vi "Axial.vi"() -> ()   [LabVIEW 2017]
uses:
  <vilib>/Analysis/Matrix/Datatypes/RealMatrix.ctl
  <vilib>/Analysis/baseanly.llb/Mean (DBL).vi
  <vilib>/ULx/Create Channel.llb/ULx Create Channel (AI-Voltage-Basic).vi
  <vilib>/ULx/Timing.llb/ULx Timing (Sample Clock).vi
  <vilib>/ULx/Read.llb/ULx Read (Analog Wfm 1Chan NSamp).vi
  <vilib>/Utility/file.llb/Write Delimited Spreadsheet (DBL).vi
  <vilib>/Analysis/Matrix/Numeric/Conversions/Array To Matrix - RA.vi
  <vilib>/Analysis/NI_AALBase.lvlib
  <vilib>/Analysis/Matrix/NI_Matrix.lvlib
panel:
  out "Axial":cluster{"Weight":dbl[], "Voltage(Axial)":dbl[]}(graph)
  out "Rolling Moment":cluster{"Weight":dbl[], "Voltage(R.M.) ":dbl[]}(graph)
  out "S.F.":cluster{"Weight":dbl[], "Voltage(S.F.)":dbl[]}(graph)
  out "P.M.":cluster{"Weight":dbl[], "Voltage(P.M.)":dbl[]}(graph)
  out "n":cluster{"Weight":dbl[], "Voltage(n)":dbl[]}(graph)
  out "Normal":cluster{"Weight":dbl[], "Voltage(Normal)":dbl[]}(graph)
  out "Main Graph":cluster{"Weight":dbl[], "Main Voltage":dbl[]}(graph)
  out "Matrix Path Indicator":path
  in  "Record Matrix Path":path
  in  "Final Matrix":T1
  out "R.M. Sample Waveform":dbl[](graph)
  out "S.F. Sample Waveform":dbl[](graph)
  out "P.M. Sample Waveform":dbl[](graph)
  out "n Sample Waveform":dbl[](graph)
  out "Axial Force Sample Waveform":dbl[](graph)
  out "Normal Force Sample Waveform":dbl[](graph)
  out "Main Voltage":dbl[](array[numeric])
  out "Current Main Channel Calibration":string
  in  "Main Channel":string(combo)
  in  "Rolling Moment Physical Channel":refnum<k21>
  in  "S.F. Physical Channel":refnum<k21>
  in  "P.M. Physical Channel":refnum<k21>
  in  "n Physical Channel":refnum<k21>
  in  "Normal Force Physical Channel":refnum<k21>
  in  "minimum value":dbl=-5.0
  in  "maximum value":dbl=5.0
  in  "samples per channel":i32=100
  in  "sample mode":i32(ring) items=["FiniteSamples", "ContinuousSamples"]
  in  "rate":dbl=5000.0
  in  "Axial Force Physical Channel":refnum<k21>
  out "Voltage(R.M.)":dbl[](array[numeric])
  out "Voltage(S.F.)":dbl[](array[numeric])
  out "Voltage(P.M.)":dbl[](array[numeric])
  out "Voltage(n)":dbl[](array[numeric])
  out "Voltage(Normal)":dbl[](array[numeric])
  in  "Sample Button":bool
  in  "Add Weight":bool
  in  "Weight to be added":dbl
  out "Voltage(Axial)":dbl[](array[numeric])
  out "Weight":dbl[](array[numeric])
  in  "Clear Table":bool
  # "Channel and Sampling Selection"
  # "Interaction Plots\n\nPlots ALL SIX voltages,"
  # "Sample Waveform Graphs\n\nPlots all the data points onto a waveform graph in one sample Cycle, to see the range of noises and determine any bias in data."
  # "Voltages from EACH Channel\nRecords data from all six channels for each sample cycle. Each number represents the mean of all values from one sample cycle recorded by one channel."
  # "Final Matrix\nThe final matrix that records the data from calibration and overwrites itself every time one calibration cycle is performed."
  # "Weight"
  # "Normal Force"
  # "Axial Force"
  # "n"
  # "P.M."
  # "S.F."
  # "Rolling Moment"
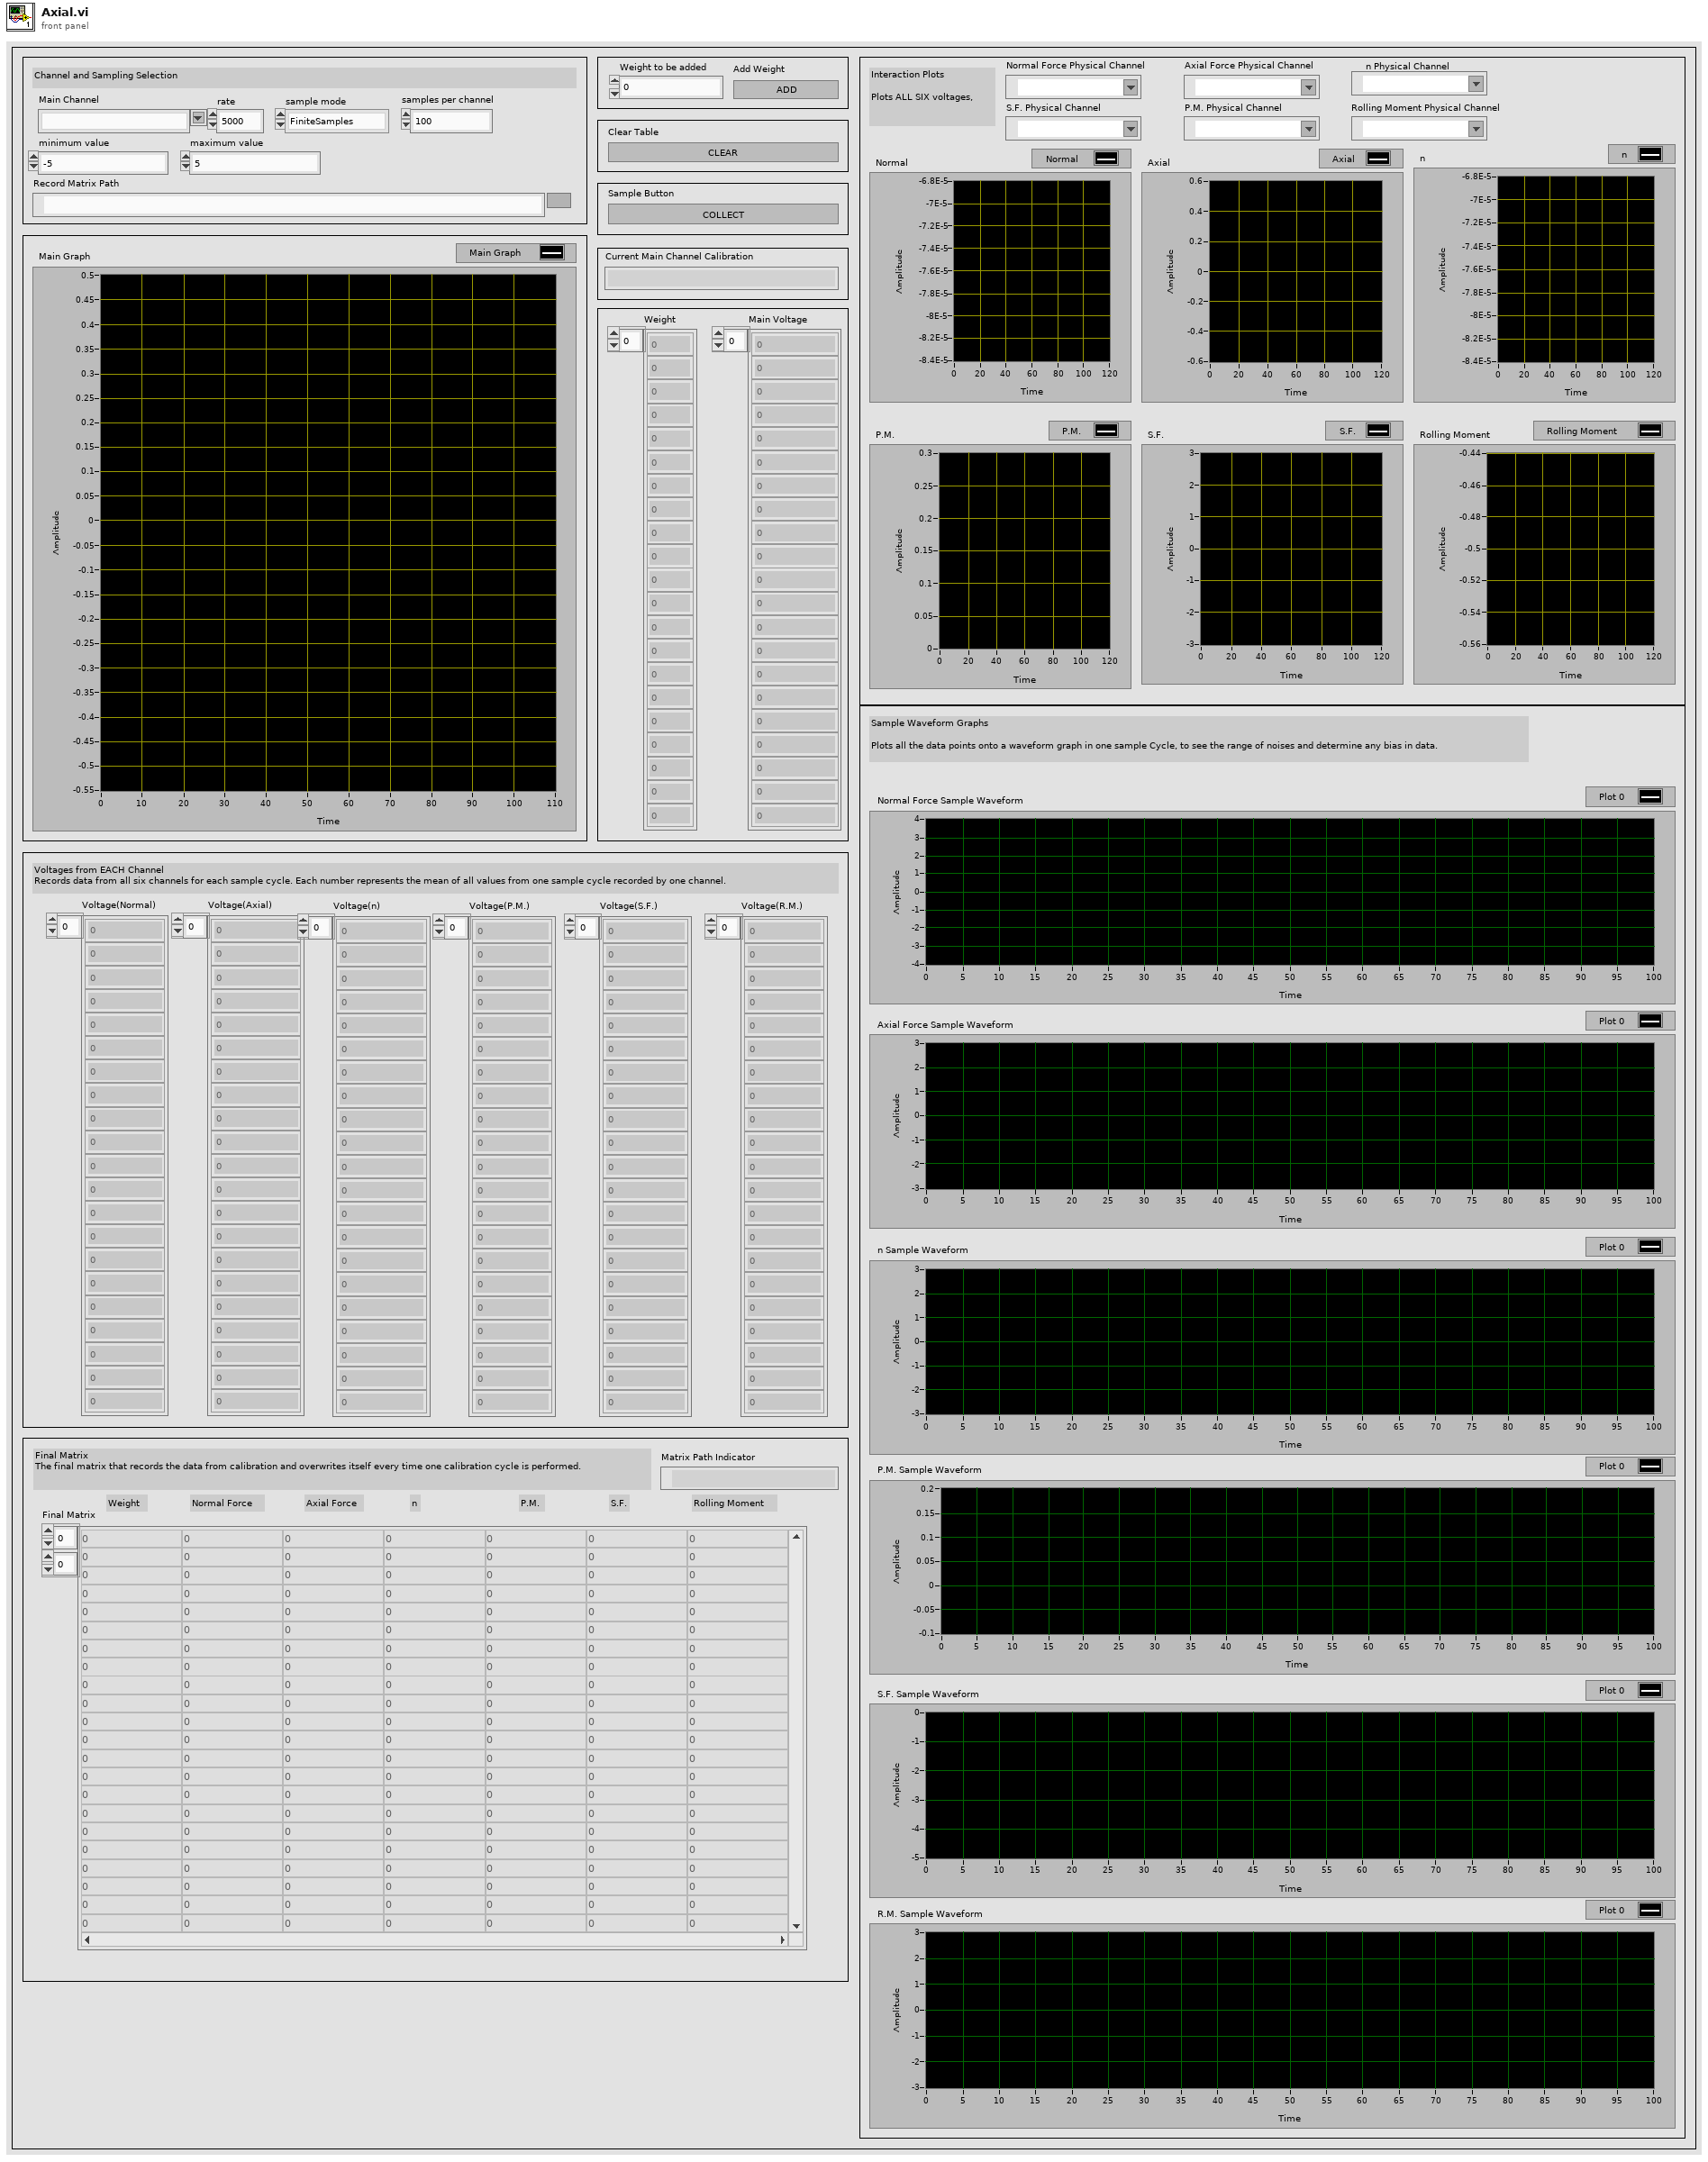
[diagram p1: front panel]
types:
  T1 = typedef "NI_Matrix.lvlib/RealMatrix.ctl" = dbl[][]
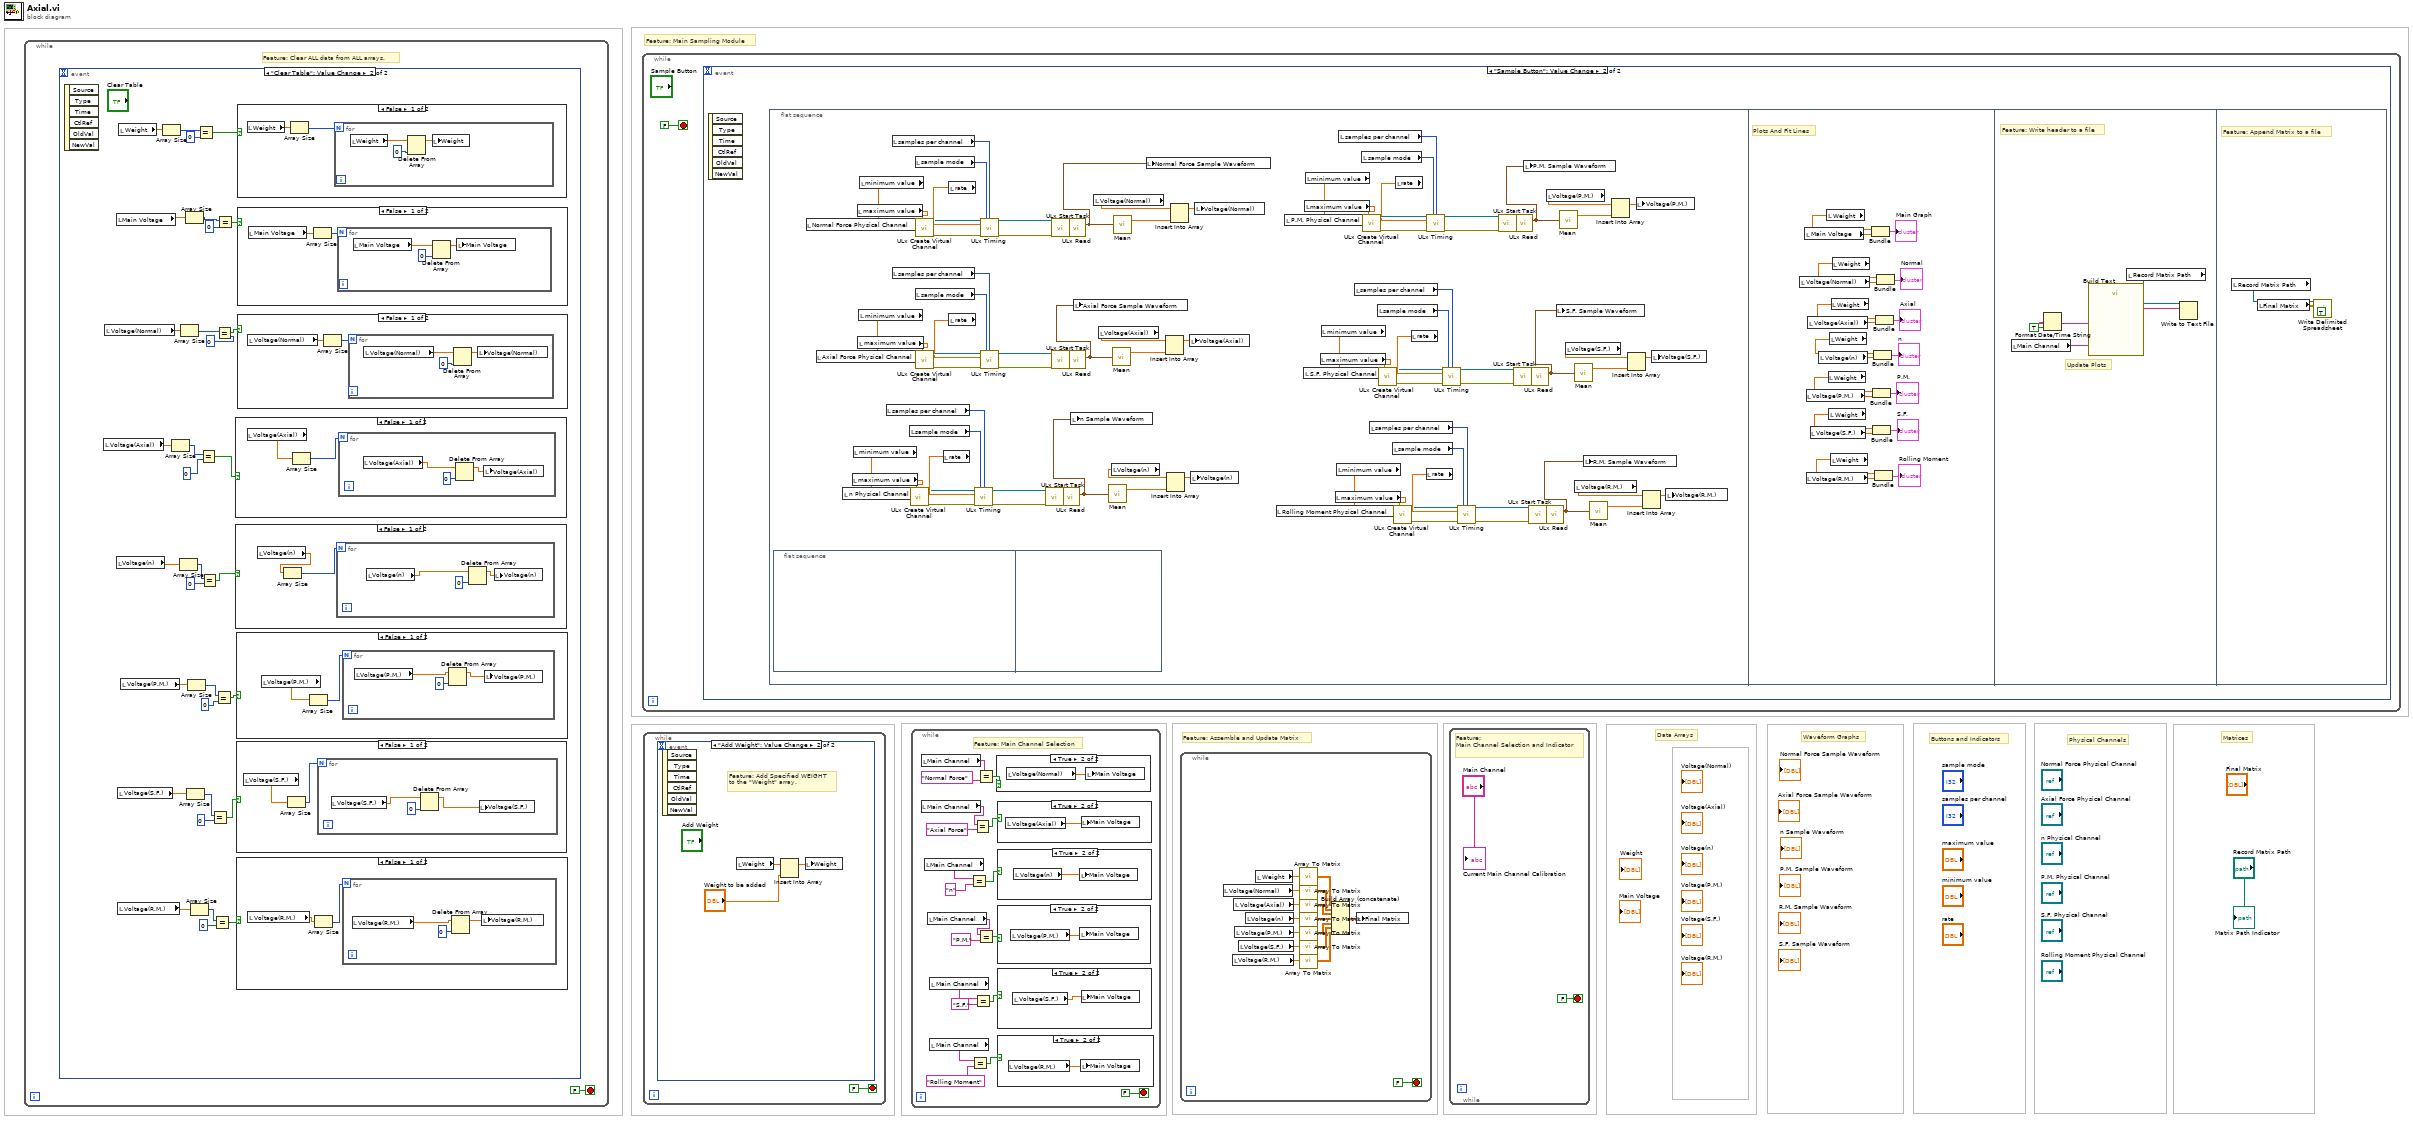
[diagram p0: block diagram]
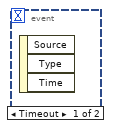
[diagram p8: hidden frame]
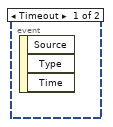
[diagram p17: hidden frame]
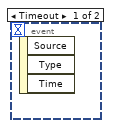
[diagram p18: hidden frame]
diagram:
  # "Matrices"
  # "Feature: Assemble and Update Matrix"
  # "Waveform Graphs"
  # "Physical Channels"
  # "Feature: Main Sampling Module"
  # "Data Arrays"
  # "Buttons and Indicators"
  n1 = while {
    stop <- FALSE stop-if-true
    # "Feature: Clear ALL data from ALL arrays."
    n2 = event shown="[1] \"Clear Table\": Value Change" {
      selector: _ -> [_ _]
      dyn-events: _ -> [_ _]
      timeout: _ -> [_ _]
      event Timeout {
        n3 = event-data() -> ()  [unwired: 1 in, 3 out]
      }
      event "Clear Table": Value Change {
        n4 = event-data() -> ()  [unwired: 1 in, 6 out]
        n5 = local read "Voltage(Axial)"() -> (w21:dbl[])
        n6 = local read "Voltage(Normal)"() -> (w24:dbl[])
        n7 = local read "Main Voltage"() -> (w30:dbl[])
        n8 = local read "Voltage(n)"() -> (w18:dbl[])
        n9 = local read "Voltage(S.F.)"() -> (w10:dbl[])
        n10 = local read "Voltage(R.M.)"() -> (w6:dbl[])
        n11 = local read "Weight"() -> (w31:dbl[])
        n12 = local read "Voltage(P.M.)"() -> (w13:dbl[])
        n13 = Array Size(array=w31) -> (size(s)=w34:i32)
        n14 = Array Size(array=w21) -> (size(s)=w22:i32)
        n15 = Array Size(array=w18) -> (size(s)=w17:i32)
        n16 = Array Size(array=w24) -> (size(s)=w25:i32)
        n17 = Array Size(array=w30) -> (size(s)=w29:i32)
        n18 = Array Size(array=w10) -> (size(s)=w9:i32)
        n19 = Array Size(array=w13) -> (size(s)=w14:i32)
        n20 = Array Size(array=w6) -> (size(s)=w5:i32)
        n21 = Equal?(x=w34, y=0) -> (x = y?=w32:bool)
        n22 = Equal?(x=w22, y=0) -> (x = y?=w19:bool)
        n23 = Equal?(x=w17, y=0) -> (x = y?=w15:bool)
        n24 = Equal?(x=w9, y=0) -> (x = y?=w7:bool)
        n25 = Equal?(x=w5, y=0) -> (x = y?=w4:bool)
        n26 = Equal?(x=w14, y=0) -> (x = y?=w11:bool)
        n27 = Equal?(x=w25, y=0) -> (x = y?=w26:bool)
        n28 = Equal?(x=w29, y=0) -> (x = y?=w27:bool)
        n29 = case shown="False" w19 {
          frame False {
            n30 = local read "Voltage(Axial)"() -> (w56:dbl[])
            n31 = Array Size(array=w56) -> (size(s)=w55:i32)
            n32 = for {
              N: w55 -> [_]
              n33 = local read "Voltage(Axial)"() -> (w59:dbl[])
              n34 = Delete From Array(array=w59, index=0) -> (array with subset deleted=w57:dbl[])  [unwired: 1 in, 1 out]
              n35 = local write "Voltage(Axial)"(w57) -> ()
            }
          }
          frame True {
          }
        }
        n36 = case shown="False" w15 {
          frame False {
            n37 = local read "Voltage(n)"() -> (w51:dbl[])
            n38 = Array Size(array=w51) -> (size(s)=w50:i32)
            n39 = for {
              N: w50 -> [_]
              n40 = local read "Voltage(n)"() -> (w54:dbl[])
              n41 = Delete From Array(array=w54, index=0) -> (array with subset deleted=w52:dbl[])  [unwired: 1 in, 1 out]
              n42 = local write "Voltage(n)"(w52) -> ()
            }
          }
          frame True {
          }
        }
        n43 = case shown="False" w11 {
          frame False {
            n44 = local read "Voltage(P.M.)"() -> (w46:dbl[])
            n45 = Array Size(array=w46) -> (size(s)=w45:i32)
            n46 = for {
              N: w45 -> [_]
              n47 = local read "Voltage(P.M.)"() -> (w49:dbl[])
              n48 = Delete From Array(array=w49, index=0) -> (array with subset deleted=w47:dbl[])  [unwired: 1 in, 1 out]
              n49 = local write "Voltage(P.M.)"(w47) -> ()
            }
          }
          frame True {
          }
        }
        n50 = case shown="False" w7 {
          frame False {
            n51 = local read "Voltage(S.F.)"() -> (w41:dbl[])
            n52 = Array Size(array=w41) -> (size(s)=w40:i32)
            n53 = for {
              N: w40 -> [_]
              n54 = local read "Voltage(S.F.)"() -> (w44:dbl[])
              n55 = Delete From Array(array=w44, index=0) -> (array with subset deleted=w43:dbl[])  [unwired: 1 in, 1 out]
              n56 = local write "Voltage(S.F.)"(w43) -> ()
            }
          }
          frame True {
          }
        }
        n57 = case shown="False" w4 {
          frame False {
            n58 = local read "Voltage(R.M.)"() -> (w35:dbl[])
            n59 = Array Size(array=w35) -> (size(s)=w36:i32)
            n60 = for {
              N: w36 -> [_]
              n61 = local read "Voltage(R.M.)"() -> (w39:dbl[])
              n62 = Delete From Array(array=w39, index=0) -> (array with subset deleted=w37:dbl[])  [unwired: 1 in, 1 out]
              n63 = local write "Voltage(R.M.)"(w37) -> ()
            }
          }
          frame True {
          }
        }
        n64 = case shown="False" w26 {
          frame False {
            n65 = local read "Voltage(Normal)"() -> (w61:dbl[])
            n66 = Array Size(array=w61) -> (size(s)=w60:i32)
            n67 = for {
              N: w60 -> [_]
              n68 = local read "Voltage(Normal)"() -> (w64:dbl[])
              n69 = Delete From Array(array=w64, index=0) -> (array with subset deleted=w63:dbl[])  [unwired: 1 in, 1 out]
              n70 = local write "Voltage(Normal)"(w63) -> ()
            }
          }
          frame True {
          }
        }
        n71 = case shown="False" w32 {
          frame False {
            n72 = local read "Weight"() -> (w71:dbl[])
            n73 = Array Size(array=w71) -> (size(s)=w70:i32)
            n74 = for {
              N: w70 -> [_]
              n75 = local read "Weight"() -> (w73:dbl[])
              n76 = Delete From Array(array=w73, index=0) -> (array with subset deleted=w72:dbl[])  [unwired: 1 in, 1 out]
              n77 = local write "Weight"(w72) -> ()
            }
          }
          frame True {
          }
        }
        n78 = case shown="False" w27 {
          frame False {
            n79 = local read "Main Voltage"() -> (w66:dbl[])
            n80 = Array Size(array=w66) -> (size(s)=w65:i32)
            n81 = for {
              N: w65 -> [_]
              n82 = local read "Main Voltage"() -> (w68:dbl[])
              n83 = Delete From Array(array=w68, index=0) -> (array with subset deleted=w69:dbl[])  [unwired: 1 in, 1 out]
              n84 = local write "Main Voltage"(w69) -> ()
            }
          }
          frame True {
          }
        }
      }
    }
  }
  n85 = while {
    stop <- FALSE stop-if-true
    n86 = event shown="[1] \"Sample Button\": Value Change" {
      selector: _ -> [_ _]
      dyn-events: _ -> [_ _]
      timeout: _ -> [_ _]
      event Timeout {
        n87 = event-data() -> ()  [unwired: 1 in, 3 out]
      }
      event "Sample Button": Value Change {
        n88 = event-data() -> ()  [unwired: 1 in, 6 out]
        n89 = flat-sequence {
          frame #0 {
            n90 = local read "Normal Force Physical Channel"() -> (w156:refnum<k21>)
            n91 = local read "Axial Force Physical Channel"() -> (w157:refnum<k21>)
            n92 = local read "n Physical Channel"() -> (w141:refnum<k21>)
            n93 = local read "maximum value"() -> (w137:dbl)
            n94 = local read "minimum value"() -> (w136:dbl)
            n95 = local read "maximum value"() -> (w154:dbl)
            n96 = local read "maximum value"() -> (w161:dbl)
            n97 = local read "minimum value"() -> (w168:dbl)
            n98 = local read "minimum value"() -> (w155:dbl)
            n99 = local read "samples per channel"() -> (w139:i32)
            n100 = local read "samples per channel"() -> (w150:i32)
            n101 = local read "samples per channel"() -> (w158:i32)
            n102 = local read "sample mode"() -> (w138:i32)
            n103 = call-poly <vilib>:"ULx Create Virtual Channel.vi"("maximum value"=w137, "minimum value"=w136, "physical channels"=w141) -> ("task out"=w127:refnum<k24>, "error out"=w128:errorcluster)  [unwired: 11 in]
            n104 = local read "sample mode"() -> (w151:i32)
            n105 = local read "sample mode"() -> (w159:i32)
            n106 = call-poly <vilib>:"ULx Create Virtual Channel.vi"("maximum value"=w154, "minimum value"=w155, "physical channels"=w156) -> ("task out"=w149:refnum<k24>, "error out"=w153:errorcluster)  [unwired: 11 in]
            n107 = call-poly <vilib>:"ULx Create Virtual Channel.vi"("maximum value"=w161, "minimum value"=w168, "physical channels"=w157) -> ("task out"=w162:refnum<k24>, "error out"=w167:errorcluster)  [unwired: 11 in]
            n108 = local read "rate"() -> (w140:dbl)
            n109 = local read "rate"() -> (w152:dbl)
            n110 = local read "rate"() -> (w160:dbl)
            n111 = call-poly <vilib>:"ULx Timing.vi"("task in"=w127, "sample mode"=w138, "samples per channel"=w139, "rate"=w140, "error in"=w128) -> ("task out"=w130:refnum<k24>, "error out"=w129:errorcluster)  [unwired: 9 in]
            n112 = call-poly <vilib>:"ULx Timing.vi"("task in"=w149, "sample mode"=w151, "samples per channel"=w150, "rate"=w152, "error in"=w153) -> ("task out"=w148:refnum<k24>, "error out"=w147:errorcluster)  [unwired: 9 in]
            n113 = call-poly <vilib>:"ULx Timing.vi"("task in"=w162, "sample mode"=w159, "samples per channel"=w158, "rate"=w160, "error in"=w167) -> ("task out"=w163:refnum<k24>, "error out"=w166:errorcluster)  [unwired: 9 in]
            n114 = call <vilib>:"ULx Start Task.vi"("task in"=w130, "error in"=w129) -> ("task out"=w132:refnum<k24>, "error out"=w131:errorcluster)  [unwired: 12 in]
            n115 = call <vilib>:"ULx Start Task.vi"("task in"=w148, "error in"=w147) -> ("task out"=w146:refnum<k24>, "error out"=w145:errorcluster)  [unwired: 12 in]
            n116 = call <vilib>:"ULx Start Task.vi"("task in"=w163, "error in"=w166) -> ("task out"=w164:refnum<k24>, "error out"=w165:errorcluster)  [unwired: 12 in]
            n117 = call-poly <vilib>:"ULx Read.vi"("task in"=w132, "error in"=w131) -> ("data"=w79:waveform(dbl))  [unwired: 11 in, 2 out]
            n118 = call-poly <vilib>:"ULx Read.vi"("task in"=w146, "error in"=w145) -> ("data"=w81:waveform(dbl))  [unwired: 11 in, 2 out]
            n119 = call-poly <vilib>:"ULx Read.vi"("task in"=w164, "error in"=w165) -> ("data"=w80:waveform(dbl))  [unwired: 11 in, 2 out]
            n120 = local write "n Sample Waveform"(w79) -> ()
            n121 = local write "Axial Force Sample Waveform"(w80) -> ()
            n122 = local read "Voltage(Normal)"() -> (w143:dbl[])
            n123 = local read "Voltage(Axial)"() -> (w170:dbl[])
            n124 = call-poly <vilib>:"Mean.vi"("X"=w79) -> ("mean"=w133:dbl)  [unwired: 1 out]
            n125 = local read "Voltage(n)"() -> (w135:dbl[])
            n126 = call-poly <vilib>:"Mean.vi"("X"=w80) -> ("mean"=w169:dbl)  [unwired: 1 out]
            n127 = call-poly <vilib>:"Mean.vi"("X"=w81) -> ("mean"=w144:dbl)  [unwired: 1 out]
            n128 = local write "Normal Force Sample Waveform"(w81) -> ()
            n129 = Insert Into Array(array=w170, new element=w169) -> (w171:dbl[])  [unwired: 1 in]
            n130 = Insert Into Array(array=w135, new element=w133) -> (w134:dbl[])  [unwired: 1 in]
            n131 = Insert Into Array(array=w143, new element=w144) -> (w142:dbl[])  [unwired: 1 in]
            n132 = local write "Voltage(Axial)"(w171) -> ()
            n133 = local write "Voltage(n)"(w134) -> ()
            n134 = local write "Voltage(Normal)"(w142) -> ()
            n135 = local read "Rolling Moment Physical Channel"() -> (w100:refnum<k21>)
            n136 = local read "P.M. Physical Channel"() -> (w126:refnum<k21>)
            n137 = local read "S.F. Physical Channel"() -> (w101:refnum<k21>)
            n138 = local read "maximum value"() -> (w125:dbl)
            n139 = local read "minimum value"() -> (w124:dbl)
            n140 = local read "maximum value"() -> (w98:dbl)
            n141 = local read "minimum value"() -> (w99:dbl)
            n142 = local read "maximum value"() -> (w86:dbl)
            n143 = local read "minimum value"() -> (w87:dbl)
            n144 = local read "samples per channel"() -> (w116:i32)
            n145 = local read "samples per channel"() -> (w95:i32)
            n146 = local read "sample mode"() -> (w115:i32)
            n147 = call-poly <vilib>:"ULx Create Virtual Channel.vi"("maximum value"=w125, "minimum value"=w124, "physical channels"=w126) -> ("task out"=w123:refnum<k24>, "error out"=w114:errorcluster)  [unwired: 11 in]
            n148 = local read "samples per channel"() -> (w89:i32)
            n149 = local read "sample mode"() -> (w94:i32)
            n150 = call-poly <vilib>:"ULx Create Virtual Channel.vi"("maximum value"=w98, "minimum value"=w99, "physical channels"=w101) -> ("task out"=w97:refnum<k24>, "error out"=w96:errorcluster)  [unwired: 11 in]
            n151 = local read "sample mode"() -> (w88:i32)
            n152 = call-poly <vilib>:"ULx Create Virtual Channel.vi"("maximum value"=w86, "minimum value"=w87, "physical channels"=w100) -> ("task out"=w85:refnum<k24>, "error out"=w84:errorcluster)  [unwired: 11 in]
            n153 = local read "rate"() -> (w122:dbl)
            n154 = local read "rate"() -> (w121:dbl)
            n155 = local read "rate"() -> (w120:dbl)
            n156 = call-poly <vilib>:"ULx Timing.vi"("task in"=w123, "sample mode"=w115, "samples per channel"=w116, "rate"=w122, "error in"=w114) -> ("task out"=w113:refnum<k24>, "error out"=w112:errorcluster)  [unwired: 9 in]
            n157 = call-poly <vilib>:"ULx Timing.vi"("task in"=w97, "sample mode"=w94, "samples per channel"=w95, "rate"=w121, "error in"=w96) -> ("task out"=w93:refnum<k24>, "error out"=w92:errorcluster)  [unwired: 9 in]
            n158 = call-poly <vilib>:"ULx Timing.vi"("task in"=w85, "sample mode"=w88, "samples per channel"=w89, "rate"=w120, "error in"=w84) -> ("task out"=w83:refnum<k24>, "error out"=w82:errorcluster)  [unwired: 9 in]
            n159 = call <vilib>:"ULx Start Task.vi"("task in"=w113, "error in"=w112) -> ("task out"=w111:refnum<k24>, "error out"=w110:errorcluster)  [unwired: 12 in]
            n160 = call <vilib>:"ULx Start Task.vi"("task in"=w93, "error in"=w92) -> ("task out"=w91:refnum<k24>, "error out"=w90:errorcluster)  [unwired: 12 in]
            n161 = call-poly <vilib>:"ULx Read.vi"("task in"=w111, "error in"=w110) -> ("data"=w77:waveform(dbl))  [unwired: 11 in, 2 out]
            n162 = local write "P.M. Sample Waveform"(w77) -> ()
            n163 = call <vilib>:"ULx Start Task.vi"("task in"=w83, "error in"=w82) -> ("task out"=w106:refnum<k24>, "error out"=w105:errorcluster)  [unwired: 12 in]
            n164 = call-poly <vilib>:"ULx Read.vi"("task in"=w91, "error in"=w90) -> ("data"=w76:waveform(dbl))  [unwired: 11 in, 2 out]
            n165 = call-poly <vilib>:"ULx Read.vi"("task in"=w106, "error in"=w105) -> ("data"=w78:waveform(dbl))  [unwired: 11 in, 2 out]
            n166 = local read "Voltage(P.M.)"() -> (w118:dbl[])
            n167 = local write "S.F. Sample Waveform"(w76) -> ()
            n168 = call-poly <vilib>:"Mean.vi"("X"=w77) -> ("mean"=w119:dbl)  [unwired: 1 out]
            n169 = local read "Voltage(S.F.)"() -> (w103:dbl[])
            n170 = call-poly <vilib>:"Mean.vi"("X"=w76) -> ("mean"=w104:dbl)  [unwired: 1 out]
            n171 = local read "Voltage(R.M.)"() -> (w108:dbl[])
            n172 = local write "R.M. Sample Waveform"(w78) -> ()
            n173 = call-poly <vilib>:"Mean.vi"("X"=w78) -> ("mean"=w107:dbl)  [unwired: 1 out]
            n174 = Insert Into Array(array=w118, new element=w119) -> (w117:dbl[])  [unwired: 1 in]
            n175 = Insert Into Array(array=w103, new element=w104) -> (w102:dbl[])  [unwired: 1 in]
            n176 = local write "Voltage(P.M.)"(w117) -> ()
            n177 = Insert Into Array(array=w108, new element=w107) -> (w109:dbl[])  [unwired: 1 in]
            n178 = local write "Voltage(S.F.)"(w102) -> ()
            n179 = local write "Voltage(R.M.)"(w109) -> ()
          }
          frame #1 {
            # "Plots And Fit Lines"
            n180 = local read "Voltage(Normal)"() -> (w188:dbl[])
            n181 = local read "Main Voltage"() -> (w191:dbl[])
            n182 = local read "Voltage(P.M.)"() -> (w180:dbl[])
            n183 = local read "Voltage(R.M.)"() -> (w174:dbl[])
            n184 = local read "Voltage(Axial)"() -> (w185:dbl[])
            n185 = local read "Voltage(S.F.)"() -> (w177:dbl[])
            n186 = local read "Voltage(n)"() -> (w183:dbl[])
            n187 = local read "Weight"() -> (w192:dbl[])
            n188 = local read "Weight"() -> (w181:dbl[])
            n189 = local read "Weight"() -> (w178:dbl[])
            n190 = local read "Weight"() -> (w184:dbl[])
            n191 = local read "Weight"() -> (w175:dbl[])
            n192 = local read "Weight"() -> (w186:dbl[])
            n193 = local read "Weight"() -> (w189:dbl[])
            n194 = Bundle("Weight"=w192, "Main Voltage"=w191) -> (→"Main Graph":cluster{"Weight":dbl[], "Main Voltage":dbl[]})  [unwired: 1 in]
            n195 = Bundle("Weight"=w181, "Voltage(P.M.)"=w180) -> (→"P.M.":cluster{"Weight":dbl[], "Voltage(P.M.)":dbl[]})  [unwired: 1 in]
            n196 = Bundle("Weight"=w178, "Voltage(S.F.)"=w177) -> (→"S.F.":cluster{"Weight":dbl[], "Voltage(S.F.)":dbl[]})  [unwired: 1 in]
            n197 = Bundle("Weight"=w184, "Voltage(n)"=w183) -> (→"n":cluster{"Weight":dbl[], "Voltage(n)":dbl[]})  [unwired: 1 in]
            n198 = Bundle("Weight"=w175, "Voltage(R.M.)"=w174) -> (→"Rolling Moment":cluster{"Weight":dbl[], "Voltage(R.M.) ":dbl[]})  [unwired: 1 in]
            n199 = Bundle("Weight"=w186, "Voltage(Axial)"=w185) -> (→"Axial":cluster{"Weight":dbl[], "Voltage(Axial)":dbl[]})  [unwired: 1 in]
            n200 = Bundle("Weight"=w189, "Voltage(Normal)"=w188) -> (→"Normal":cluster{"Weight":dbl[], "Voltage(Normal)":dbl[]})  [unwired: 1 in]
          }
          frame #2 {
            # "Feature: Write header to a file"
            # "Update Plots"
            n201 = local read "Main Channel"() -> (w194:string)
            n202 = Format Date/Time String(UTC format=TRUE) -> (date/time string=w196:string)  [unwired: 2 in]
            n203 = call "Build Text"("date"=w196, "mainchannel"=w194) -> ("Result"=w195:string)  [unwired: 12 in, 1 out]
            n204 = local read "Record Matrix Path"() -> (w197:path)
            n205 = Write to Text File(file (use dialog)=w197, text=w195) -> ()  [unwired: 2 in, 3 out]
          }
          frame #3 {
            # "Feature: Append Matrix to a file"
            n206 = local read "Record Matrix Path"() -> (w199:path)
            n207 = local read "Final Matrix"() -> (w200:T1)
            n208 = call-poly <vilib>:"Write Delimited Spreadsheet.vi"("file path (dialog if empty)"=w199, "2D data"=w200, "append to file? (new file:F)"=TRUE) -> ()  [unwired: 11 in, 2 out]
          }
        }
        n209 = flat-sequence {
          frame #0 {
          }
          frame #1 {
          }
        }
      }
    }
  }
  n210 = while {
    stop <- FALSE stop-if-true
    n211 = event shown="[1] \"Add Weight\": Value Change" {
      selector: _ -> [_ _]
      dyn-events: _ -> [_ _]
      timeout: _ -> [_ _]
      event Timeout {
        n212 = event-data() -> ()  [unwired: 1 in, 3 out]
      }
      event "Add Weight": Value Change {
        # "Feature: Add Specified WEIGHT\nto the \"Weight\" array."
        n213 = event-data() -> ()  [unwired: 1 in, 6 out]
        n214 = local read "Weight"() -> (w203:dbl[])
        n215 = Insert Into Array(array=w203, new element="Weight to be added") -> (w202:dbl[])  [unwired: 1 in]
        n216 = local write "Weight"(w202) -> ()
      }
    }
  }
  n217 = while {
    stop <- FALSE stop-if-true
    # "Feature: Main Channel Selection"
    n218 = local read "Main Channel"() -> (w219:string)
    n219 = local read "Main Channel"() -> (w222:string)
    n220 = local read "Main Channel"() -> (w215:string)
    n221 = local read "Main Channel"() -> (w213:string)
    n222 = local read "Main Channel"() -> (w211:string)
    n223 = local read "Main Channel"() -> (w209:string)
    n224 = Equal?(x=w215, y="n") -> (x = y?=w216:bool)
    n225 = Equal?(x=w209, y="Rolling Moment") -> (x = y?=w210:bool)
    n226 = Equal?(x=w219, y="Axial Force") -> (x = y?=w218:bool)
    n227 = Equal?(x=w211, y="S.F.") -> (x = y?=w212:bool)
    n228 = Equal?(x=w222, y="Normal Force") -> (x = y?=w220:bool)
    n229 = Equal?(x=w213, y="P.M.") -> (x = y?=w214:bool)
    n230 = case shown="True" w220 {
      frame False {
      }
      frame True {
        n231 = local read "Voltage(Normal)"() -> (w229:dbl[])
        n232 = local write "Main Voltage"(w229) -> ()
      }
    }
    n233 = case shown="True" w218 {
      frame False {
      }
      frame True {
        n234 = local read "Voltage(Axial)"() -> (w228:dbl[])
        n235 = local write "Main Voltage"(w228) -> ()
      }
    }
    n236 = case shown="True" w216 {
      frame False {
      }
      frame True {
        n237 = local read "Voltage(n)"() -> (w227:dbl[])
        n238 = local write "Main Voltage"(w227) -> ()
      }
    }
    n239 = case shown="True" w214 {
      frame False {
      }
      frame True {
        n240 = local read "Voltage(P.M.)"() -> (w226:dbl[])
        n241 = local write "Main Voltage"(w226) -> ()
      }
    }
    n242 = case shown="True" w212 {
      frame False {
      }
      frame True {
        n243 = local read "Voltage(S.F.)"() -> (w225:dbl[])
        n244 = local write "Main Voltage"(w225) -> ()
      }
    }
    n245 = case shown="True" w210 {
      frame False {
      }
      frame True {
        n246 = local read "Voltage(R.M.)"() -> (w224:dbl[])
        n247 = local write "Main Voltage"(w224) -> ()
      }
    }
  }
  n248 = while {
    stop <- FALSE stop-if-true
    n249 = local read "Voltage(Normal)"() -> (w243:dbl[])
    n250 = local read "Voltage(R.M.)"() -> (w236:dbl[])
    n251 = local read "Voltage(Axial)"() -> (w240:dbl[])
    n252 = local read "Voltage(P.M.)"() -> (w238:dbl[])
    n253 = local read "Voltage(S.F.)"() -> (w237:dbl[])
    n254 = local read "Voltage(n)"() -> (w239:dbl[])
    n255 = local read "Weight"() -> (w241:dbl[])
    n256 = call-poly <vilib>:"Array To Matrix.vi"("Real 1D Array"=w241) -> ("Real Matrix (Column Vector)"=w242:T1)
    n257 = call-poly <vilib>:"Array To Matrix.vi"("Real 1D Array"=w243) -> ("Real Matrix (Column Vector)"=w244:T1)
    n258 = call-poly <vilib>:"Array To Matrix.vi"("Real 1D Array"=w240) -> ("Real Matrix (Column Vector)"=w235:T1)
    n259 = call-poly <vilib>:"Array To Matrix.vi"("Real 1D Array"=w239) -> ("Real Matrix (Column Vector)"=w234:T1)
    n260 = call-poly <vilib>:"Array To Matrix.vi"("Real 1D Array"=w238) -> ("Real Matrix (Column Vector)"=w233:T1)
    n261 = call-poly <vilib>:"Array To Matrix.vi"("Real 1D Array"=w237) -> ("Real Matrix (Column Vector)"=w232:T1)
    n262 = call-poly <vilib>:"Array To Matrix.vi"("Real 1D Array"=w236) -> ("Real Matrix (Column Vector)"=w231:T1)
    n263 = Build Array (concatenate)(w242, w244, w235, w234, w233, w232, w231) -> (w230:T1)
    n264 = local write "Final Matrix"(w230) -> ()
  }
  n265 = while {
    stop <- FALSE stop-if-true
    # "Feature:\nMain Channel Selection and Indicator"
    "Current Main Channel Calibration" <- "Main Channel"
  }
  "Matrix Path Indicator" <- "Record Matrix Path"
